vi "Update Role Map.vi"(8 "error in (no error)":errorcluster, 9 "Role":T1, 10 "Name":string, 11 "Coffee Shop In":refnum<class "Coffee Shop.lvclass">) -> (0 "error out":errorcluster, 2 "Result Message":string, 3 "Coffee Shop Out":refnum<class "Coffee Shop.lvclass">)   [LabVIEW 2020, in "Coffee Shop.lvclass"]
uses:
  Coffee Shop.lvclass
  Public/Roles.ctl
  Coffee Shop.lvclass/Coffee Shop.ctl
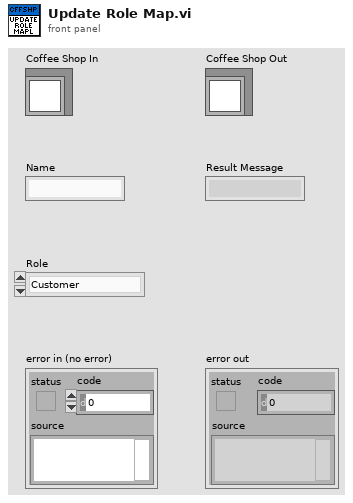
[diagram p1: front panel]
types:
  T1 = typedef "Coffee Shop.lvclass/Roles.ctl" = enum16{"Customer", "Barista", "Cashier"}
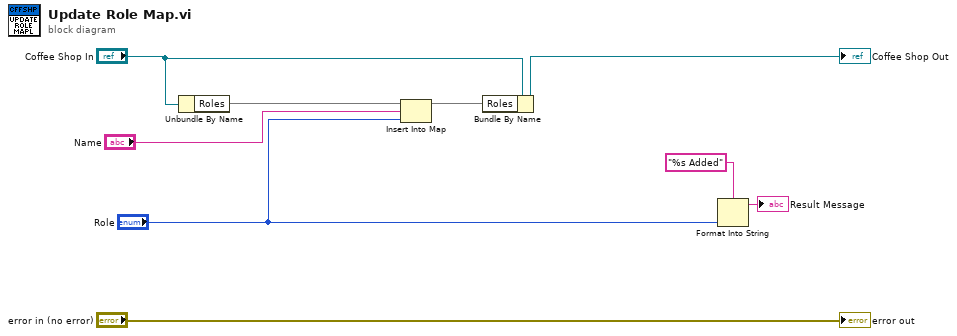
[diagram p0: block diagram]
diagram:
  n1 = Unbundle By Name("Coffee Shop In") -> ("Roles"=w8:map{string, T1})
  n2 = Insert Into Map(map in=w8, key="Name", value="Role") -> (map out=w5:map{string, T1})  [unwired: 2 out]
  n3 = Bundle By Name(cluster="Coffee Shop In", "Roles"=w5) -> (→"Coffee Shop Out":refnum<class "Coffee Shop.lvclass">)
  n4 = Format Into String(format string="%s Added", "Role") -> (resulting string=→"Result Message":string)  [unwired: 2 in, 1 out]
  "error out" <- "error in (no error)"
